vi "ServoTest.vi"() -> ()   [LabVIEW 2020]
uses:
  servoName.ctl
panel:
  in  "ServoPosition (us) 3":dbl(slide)=1500.0 scale=500.0..2500.0
  in  "Stop Button":bool
  in  "ServoPosition (us)":dbl(slide)=1500.0 scale=500.0..2500.0
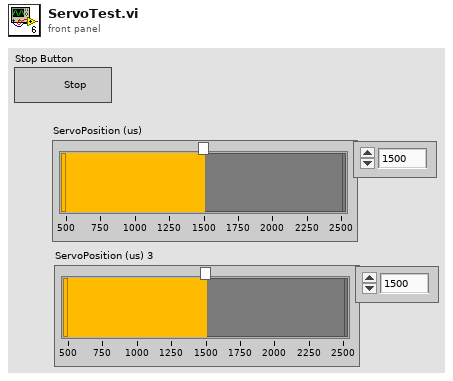
[diagram p1: front panel]
types:
  T1 = typedef "servoName.ctl" = enum16{"Servo1", "Servo2", "Servo3", "Servo4"}
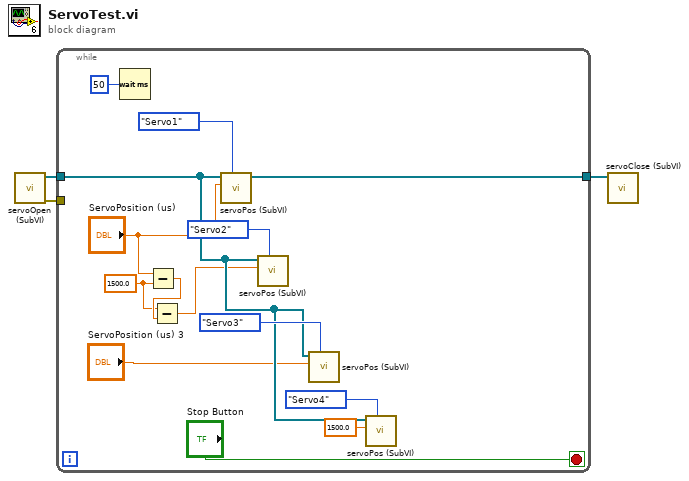
[diagram p0: block diagram]
diagram:
  n1 = call "servoOpen (SubVI).vi"() -> ("error out"=w2:errorcluster, "ServosRef"=w3:refnum<class "PWM Generator.lvclass">[])  [unwired: 10 in]
  n2 = while {
    tunnel: w3 -> [w11]
    tunnel: w2 -> [_]
    tunnel: [w14] -> w1
    stop <- "Stop Button" stop-if-true
    w6 = 1500.0 ("y")
    n3 = Wait (ms)(milliseconds to wait=u32 50) -> ()  [unwired: 1 out]
    n4 = Subtract(x="ServoPosition (us)", y=w6) -> (x-y=w7:dbl)
    n5 = Subtract(x=w6, y=w7) -> (x-y=w5:dbl)
    n6 = call "servoPos (SubVI).vi"("Servos"=servoName."Servo1", "ServoPosition (us)"="ServoPosition (us)", "ServosRef in"=w11) -> ("ServosRef out"=w14:refnum<class "PWM Generator.lvclass">[])  [unwired: 7 in, 1 out]
    n7 = call "servoPos (SubVI).vi"("Servos"=servoName."Servo2", "ServoPosition (us)"=w5, "ServosRef in"=w11) -> ()  [unwired: 7 in, 2 out]
    n8 = call "servoPos (SubVI).vi"("Servos"=servoName."Servo3", "ServoPosition (us)"="ServoPosition (us) 3", "ServosRef in"=w11) -> ()  [unwired: 7 in, 2 out]
    n9 = call "servoPos (SubVI).vi"("Servos"=servoName."Servo4", "ServoPosition (us)"=1500.0, "ServosRef in"=w11) -> ()  [unwired: 7 in, 2 out]
  }
  n10 = call "servoClose (SubVI).vi"("ServosRef"=w1) -> ()  [unwired: 10 in, 1 out]
